vi "Global LM model function and gradient (1-Exp + IRF) v2.vi"(3 "output control":T1, 4 "data":variant, 5 "X":dbl[](array[numeric]), 6 "a":dbl[](array[numeric])) -> (0 "error out":errorcluster, 1 "f'(X,a)":dbl[][](array[numeric]), 2 "f(X,a)":dbl[](array[numeric]))   [LabVIEW 2021, in "Fits.lvlib"]
doc: "This template is the starting point for creating a model function to be passed to the Nonlinear Curve Fit.vi."
uses:
  <vilib>/gmath/NumericalOptimization/LM_output select.ctl
  Graphs/XY Graph/XY Plot Data.ctl
  Global Fits/Global Fit Data.ctl
  Global Fits/Global Fit Parameters Information.ctl
  <vilib>/Analysis/2dsp.llb/1D Convolution (DBL).vi
  73fcd793-bf9d-4b1a-804b-243b66ea1503.vi
  Fits.lvlib
  <vilib>/Analysis/NI_AALPro.lvlib
  Graphs/XY Graph/XY Graph Add-Ons.lvlib
  Arrays/Arrays.lvlib
  Error/Error.lvlib
  <vilib>/gmath/NI_Gmath.lvlib
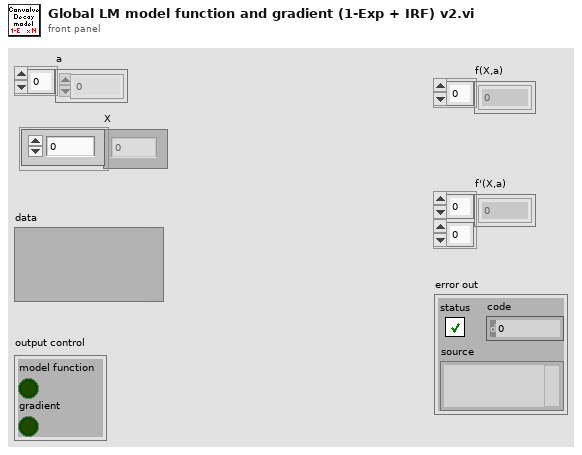
[diagram p1: front panel]
types:
  T1 = typedef "NI_Gmath.lvlib/LM_output select.ctl" = cluster{"model function":bool, "gradient":bool}
  T2 = typedef "XY Graph Add-Ons.lvlib/XY Plot Data.ctl" = cluster{"X Array":dbl[], "Y Array":dbl[]}
  T3 = typedef "Fits.lvlib/Global Fit Data.ctl" = cluster{"Fit Data":variant, "Global Fit Parameter Information":T4, "# Points in Plots":i32[]}
  T4 = typedef "Fits.lvlib/Global Fit Parameters Information.ctl" = cluster{"Original Parameter Indices":i32[], "# Global Parameters":i32, "# Plot Specific Parameters":i32, "Global Parameter? Array":bool[]}
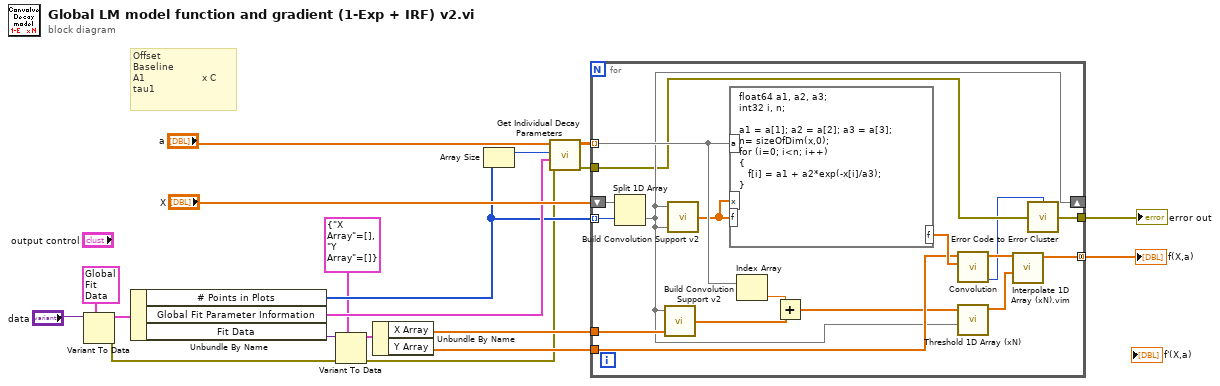
[diagram p0: block diagram]
diagram:
  # "Offset \nBaseline\nA1                   x C\ntau1"
  n1 = Variant To Data(type=T3 {"Fit Data"=variant(cluster{"t Array":dbl[], "IRF Array":dbl[]} {"t Array"=[], "IRF Array"=[]}), "Global Fit Parameter Information"={"Original Parameter Indices"=[], "# Global Parameters"=0, "# Plot Specific Parameters"=0, "Global Parameter? Array"=[]}, "# Points in Plots"=[]} ("IRF"), Variant="data") -> (data=w16:T3, error out=w5:errorcluster)  [unwired: 1 in]
  n2 = Unbundle By Name(w16) -> ("# Points in Plots"=w10:i32[], "Global Fit Parameter Information"=w11:T4, "Fit Data"=w13:variant)
  n3 = Variant To Data(error in=w5, type=T2 {"X Array"=[], "Y Array"=[]} ("Plot"), Variant=w13) -> (data=w9:T2, error out=w4:errorcluster)
  n4 = Unbundle By Name(w9) -> ("X Array"=w7:dbl[], "Y Array"=w6:dbl[])
  n5 = Array Size(array=w10) -> (size(s)=w2:i32)
  n6 = call "Get Individual Decay Parameters.vi"("Error In"=w4, "Global Fit Parameter Info"=w11, "# Decays"=w2, "Global Fit Parameters Array"="a") -> ("Error Out"=w1:errorcluster, "All Parameters Array"=w3:dbl[][])  [unwired: 4 in, 2 out]
  n7 = for {
    tunnel: w6 -> [w35]
    tunnel: w3 -> [w30] mode=indexing
    tunnel: [w24] -> w15 mode=concatenating
    tunnel: [w21] -> w14
    tunnel: w7 -> [w29]
    shift-right: [w23] -> _
    shift-left: "X" -> [w32]
    tunnel: w10 -> [w31] mode=indexing
    tunnel: w1 -> [w22]
    n8 = Split 1D Array(array=w32, index=w31) -> (second subarray=w23:dbl[])  [unwired: 1 out]
    n9 = call "Build Convolution Support v2.vi"("X Array 2"=w29, "X Array 1"=w23) -> ("X Arrays Convolution Support"=w27:dbl[])  [unwired: 3 in]
    n10 = call "Build Convolution Support v2.vi"("X Array 2"=w23, "X Array 1"=w23) -> ("X Arrays Convolution Support"=w25:dbl[])  [unwired: 3 in]
    n11 = formula code="float64 a1, a2, a3;\nint32 i, n;\n\na1 = a[1]; a2 = a[2]; a3 = a[3];\nn= sizeOfDim(x,0);\nfor (i=0; i<n; i++)\n{\n   f[i] = a1 + a2*exp(-x[i]/a3);\n}"("a"=w30, "x"=w25, "f"=w25) -> ("f"=w36:dbl[])
    n12 = Index Array(array=w30) -> (element=w28:dbl)  [unwired: 1 in]
    n13 = Add(x=w28, y=w27) -> (x+y=w26:dbl[])
    n14 = call-poly <vilib>:"Convolution.vi"("Y"=w36, "X"=w35) -> ("error"=w20:i32, "X * Y"=w34:dbl[])  [unwired: 8 in]
    n15 = call "Threshold 1D Array (xN).vi"("Search Values"=w23, "X"=w26) -> ("Interpolated Indices"=w33:dbl[])  [unwired: 9 in]
    n16 = call "Interpolate 1D Array (xN).vim"("Interpolated Indices"=w33, "Y"=w34) -> ("Interpolated Y"=w24:dbl[])  [unwired: 9 in]
    n17 = call "Error Code to Error Cluster.vi"("Error Code"=w20, "Error In"=w22) -> ("Error Out"=w21:errorcluster)  [unwired: 13 in]
  }
  "f(X,a)" <- w15
  "error out" <- w14
